vi "展开空白块.vi"(1 "索引":i32, 2 "地图":i16[][](array[numeric])) -> (0 "输出地图":i16[][](array[numeric]))   [LabVIEW 2017]
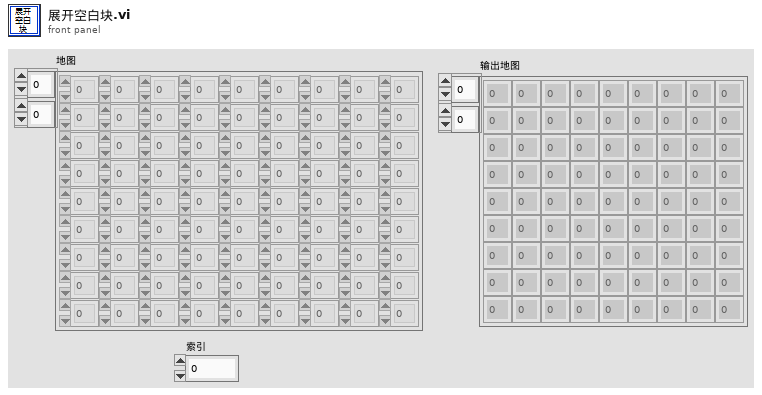
[diagram p1: front panel]
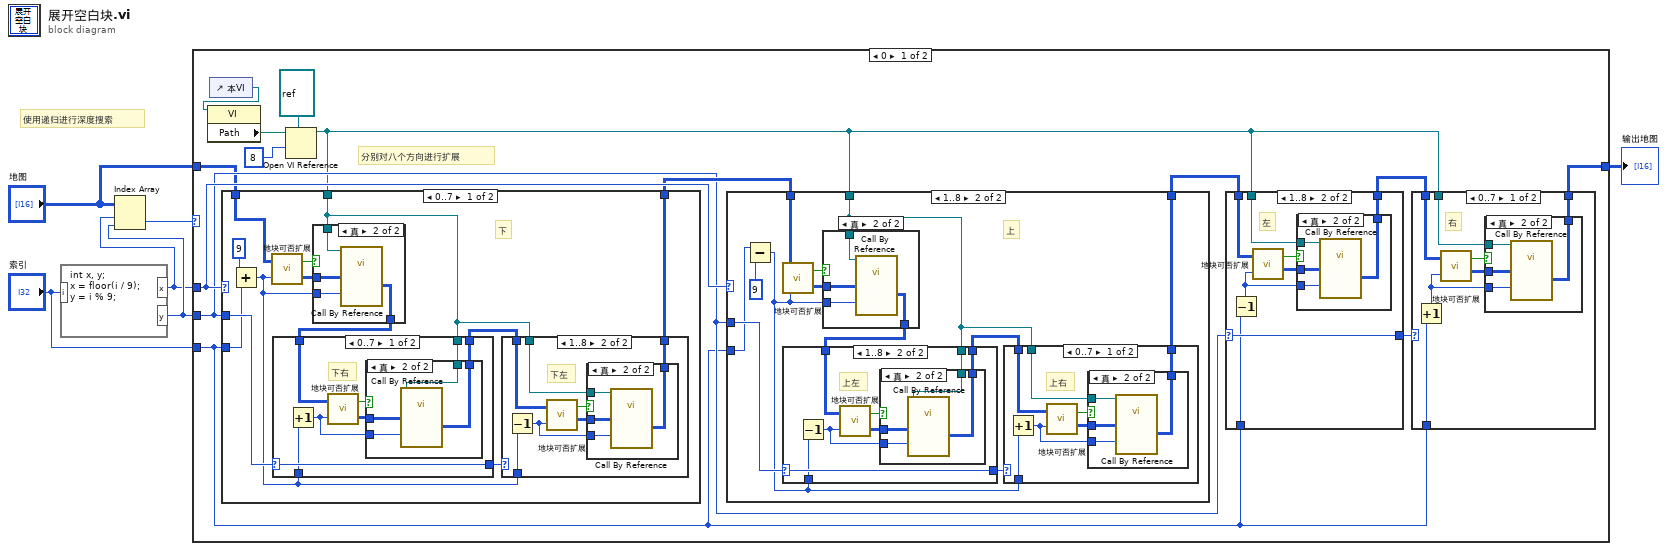
[diagram p0: block diagram]
diagram:
  # "使用递归进行深度搜索"
  n1 = formula code="int x, y;\nx = floor(i / 9);\ny = i % 9;"("i"="索引") -> ("x"=w1:i32, "y"=w2:i32)
  n2 = Index Array(array="地图", index (row)=w1, index (col)=w2) -> (element=w6:i16)
  n3 = case shown="0" w6 {
    tunnel: w1 -> [w20 _]
    tunnel: w2 -> [w18 _]
    tunnel: "索引" -> [w8 _]
    tunnel: "地图" -> [w7 w141]
    tunnel: [w14 w141] -> w3
    frame 0 {
      # "分别对八个方向进行扩展"
      n4 = control-ref of="本VI"() -> (w12:refnum<vi>)
      n5 = property class="VI"(reference=w12) -> ("Path"=w13:path)  [unwired: 1 in, 2 out]
      n6 = Open VI Reference(type specifier VI Refnum (for type only)=refnum<vi> refnum ("类型说明符VI引用句柄（仅用于类型）"), vi path=w13, options=8 ("选项")) -> (vi reference=w9:refnum<vi>)  [unwired: 3 in, 1 out]
      n7 = case shown="0..7" w20 {
        tunnel: w18 -> [w106 _]
        tunnel: w7 -> [w97 w140]
        tunnel: w8 -> [w104 _]
        tunnel: [w101 w140] -> w19
        tunnel: w9 -> [w95 _]
        frame 0..7 {
          # "下"
          n8 = Add(x=9, y=w104) -> (x+y=w96:i32)
          n9 = call "地块可否扩展.vi"("索引"=w96, "地图"=w97) -> ("输出地图"=w99:i16[][], "可展开"=w98:bool)
          n10 = case shown="真" w98 {
            tunnel: w95 -> [_ w111]
            tunnel: [w107 w110] -> w100
            tunnel: w99 -> [w107 w109]
            tunnel: w96 -> [_ w108]
            frame False {
            }
            frame True {
              n11 = call-by-ref "?"(reference=w111, "索引"=w108, "地图"=w109) -> ("输出地图"=w110:i16[][])  [unwired: 1 in, 2 out]
            }
          }
          n12 = case shown="0..7" w106 {
            selector: w106 -> [w132 w138]
            tunnel: w100 -> [w127 w139]
            tunnel: [w130 w139] -> w103
            tunnel: [w132 w138] -> w102
            tunnel: w95 -> [w131 _]
            tunnel: w96 -> [w125 _]
            frame 0..7 {
              # "下右"
              n13 = Increment(x=w125) -> (x+1=w126:i32)
              n14 = call "地块可否扩展.vi"("索引"=w126, "地图"=w127) -> ("输出地图"=w129:i16[][], "可展开"=w128:bool)
              n15 = case shown="真" w128 {
                tunnel: w131 -> [_ w137]
                tunnel: w126 -> [_ w136]
                tunnel: w129 -> [w133 w135]
                tunnel: [w133 w134] -> w130
                frame False {
                }
                frame True {
                  n16 = call-by-ref "?"(reference=w137, "索引"=w136, "地图"=w135) -> ("输出地图"=w134:i16[][])  [unwired: 1 in, 2 out]
                }
              }
            }
            frame 8, Default {
            }
          }
          n17 = case shown="1..8" w102 {
            tunnel: w103 -> [w112 w113]
            tunnel: [w112 w118] -> w101
            tunnel: w96 -> [_ w119]
            tunnel: w95 -> [_ w117]
            frame 0, Default {
            }
            frame 1..8 {
              # "下左"
              n18 = Decrement(x=w119) -> (x-1=w115:i32)
              n19 = call "地块可否扩展.vi"("索引"=w115, "地图"=w113) -> ("输出地图"=w116:i16[][], "可展开"=w114:bool)
              n20 = case shown="真" w114 {
                tunnel: w115 -> [_ w124]
                tunnel: w116 -> [w120 w123]
                tunnel: [w120 w122] -> w118
                tunnel: w117 -> [_ w121]
                frame False {
                }
                frame True {
                  n21 = call-by-ref "?"(reference=w121, "索引"=w124, "地图"=w123) -> ("输出地图"=w122:i16[][])  [unwired: 1 in, 2 out]
                }
              }
            }
          }
        }
        frame 8, Default {
        }
      }
      n22 = case shown="1..8" w20 {
        tunnel: w19 -> [w49 w52]
        tunnel: w8 -> [_ w59]
        tunnel: w18 -> [_ w61]
        tunnel: [w49 w57] -> w17
        tunnel: w9 -> [_ w50]
        frame 0, Default {
        }
        frame 1..8 {
          # "上"
          n23 = Subtract(x=w59, y=9 ("x")) -> (x-y=w51:i32)
          n24 = call "地块可否扩展.vi"("索引"=w51, "地图"=w52) -> ("输出地图"=w53:i16[][], "可展开"=w54:bool)
          n25 = case shown="真" w54 {
            tunnel: [w62 w66] -> w55
            tunnel: w50 -> [_ w65]
            tunnel: w53 -> [w62 w64]
            tunnel: w51 -> [_ w63]
            frame False {
            }
            frame True {
              n26 = call-by-ref "?"(reference=w65, "索引"=w63, "地图"=w64) -> ("输出地图"=w66:i16[][])  [unwired: 1 in, 2 out]
            }
          }
          n27 = case shown="1..8" w61 {
            selector: w61 -> [w80 w89]
            tunnel: w55 -> [w81 w83]
            tunnel: [w81 w88] -> w60
            tunnel: [w80 w89] -> w56
            tunnel: w50 -> [_ w87]
            tunnel: w51 -> [_ w82]
            frame 0, Default {
            }
            frame 1..8 {
              # "上左"
              n28 = Decrement(x=w82) -> (x-1=w84:i32)
              n29 = call "地块可否扩展.vi"("索引"=w84, "地图"=w83) -> ("输出地图"=w85:i16[][], "可展开"=w86:bool)
              n30 = case shown="真" w86 {
                tunnel: [w90 w94] -> w88
                tunnel: w87 -> [_ w93]
                tunnel: w85 -> [w90 w92]
                tunnel: w84 -> [_ w91]
                frame False {
                }
                frame True {
                  n31 = call-by-ref "?"(reference=w93, "索引"=w91, "地图"=w92) -> ("输出地图"=w94:i16[][])  [unwired: 1 in, 2 out]
                }
              }
            }
          }
          n32 = case shown="0..7" w56 {
            tunnel: w60 -> [w70 w79]
            tunnel: w51 -> [w73 _]
            tunnel: [w72 w79] -> w57
            tunnel: w50 -> [w71 _]
            frame 0..7 {
              # "上右"
              n33 = Increment(x=w73) -> (x+1=w67:i32)
              n34 = call "地块可否扩展.vi"("索引"=w67, "地图"=w70) -> ("输出地图"=w68:i16[][], "可展开"=w69:bool)
              n35 = case shown="真" w69 {
                tunnel: [w74 w78] -> w72
                tunnel: w67 -> [_ w77]
                tunnel: w71 -> [_ w76]
                tunnel: w68 -> [w74 w75]
                frame False {
                }
                frame True {
                  n36 = call-by-ref "?"(reference=w76, "索引"=w77, "地图"=w75) -> ("输出地图"=w78:i16[][])  [unwired: 1 in, 2 out]
                }
              }
            }
            frame 8, Default {
            }
          }
        }
      }
      n37 = case shown="1..8" w18 {
        selector: w18 -> [w35 w43]
        tunnel: [w35 w43] -> w16
        tunnel: w17 -> [w34 w39]
        tunnel: w8 -> [_ w42]
        tunnel: [w34 w40] -> w15
        tunnel: w9 -> [_ w41]
        frame 0, Default {
        }
        frame 1..8 {
          # "左"
          n38 = Decrement(x=w42) -> (x-1=w36:i32)
          n39 = call "地块可否扩展.vi"("索引"=w36, "地图"=w39) -> ("输出地图"=w37:i16[][], "可展开"=w38:bool)
          n40 = case shown="真" w38 {
            tunnel: w41 -> [_ w48]
            tunnel: [w44 w47] -> w40
            tunnel: w37 -> [w44 w46]
            tunnel: w36 -> [_ w45]
            frame False {
            }
            frame True {
              n41 = call-by-ref "?"(reference=w48, "索引"=w45, "地图"=w46) -> ("输出地图"=w47:i16[][])  [unwired: 1 in, 2 out]
            }
          }
        }
      }
      n42 = case shown="0..7" w16 {
        tunnel: w15 -> [w24 w33]
        tunnel: [w26 w33] -> w14
        tunnel: w8 -> [w27 _]
        tunnel: w9 -> [w25 _]
        frame 0..7 {
          # "右"
          n43 = Increment(x=w27) -> (x+1=w23:i32)
          n44 = call "地块可否扩展.vi"("索引"=w23, "地图"=w24) -> ("输出地图"=w22:i16[][], "可展开"=w21:bool)
          n45 = case shown="真" w21 {
            tunnel: [w28 w32] -> w26
            tunnel: w25 -> [_ w31]
            tunnel: w23 -> [_ w30]
            tunnel: w22 -> [w28 w29]
            frame False {
            }
            frame True {
              n46 = call-by-ref "?"(reference=w31, "索引"=w30, "地图"=w29) -> ("输出地图"=w32:i16[][])  [unwired: 1 in, 2 out]
            }
          }
        }
        frame 8, Default {
        }
      }
    }
    frame 1..8, Default {
    }
  }
  "输出地图" <- w3
